vi "niRFUtil WFM Scale Waveform (complex wfm).vi"(4 "Scaling Waveform":T1 {"y" format="%.2f"; "dx" format="%^.2e"; "x0" format="%^.2e"}, 5 "Waveform In":T1 {"y" format="%.2f"; "dx" format="%^.2e"; "x0" format="%^.2e"}) -> (2 "Waveform Out":T1 {"y" format="%.2f"; "dx" format="%^.2e"; "x0" format="%^.2e"})   [LabVIEW 2015, in "niRFUtil.lvlib"]
doc: "(c) Copyright 2006, National Instruments, Inc. This VI may not be duplicated, sold, or distributed without written consent from National Instruments."
uses:
  niRFUtil.lvlib
  Includes/niRFUtil INC Complex Waveform.ctl
  Includes/niRFUtil INC Complex Array.ctl
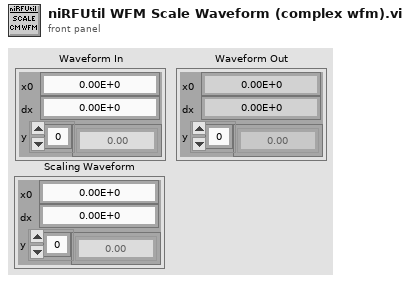
[diagram p1: front panel]
types:
  T1 = typedef "niRFUtil.lvlib/niRFUtil INC Complex Waveform.ctl" = cluster{"x0":dbl, "dx":dbl, "y":T2}
  T2 = typedef "niRFUtil.lvlib/niRFUtil INC Complex Array.ctl" = csg[]
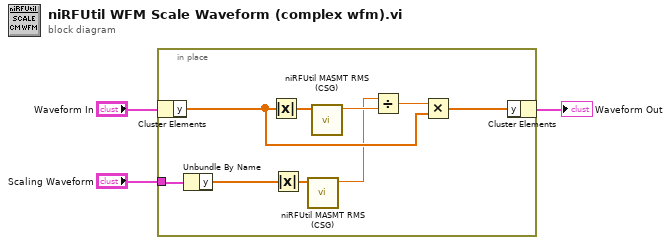
[diagram p0: block diagram]
diagram:
  n1 = in-place {
    in-place-border: "Scaling Waveform" -> [w12]
    n2 = in-place-cluster #1("Waveform In") -> ("y"=w8:T2)
    n3 = Unbundle By Name(w12) -> ("y"=w10:T2)
    n4 = Absolute Value(x=w8) -> (abs(x)=w7:sgl[])
    n5 = Absolute Value(x=w10) -> (abs(x)=w5:sgl[])
    n6 = call "niRFUtil MASMT RMS (CSG).vi"("X"=w5) -> ("rms"=w4:sgl)  [unwired: 9 in, 1 out]
    n7 = call "niRFUtil MASMT RMS (CSG).vi"("X"=w7) -> ("rms"=w6:sgl)  [unwired: 9 in, 1 out]
    n8 = Divide(x=w4, y=w6) -> (x/y=w11:sgl)
    n9 = Multiply(x=w11, y=w8) -> (x*y=w9:T2)
    n10 = in-place-cluster #1("y"=w9) -> (→"Waveform Out":T1)
  }
